vi "SHIFT REGISTER.vi"() -> ()   [LabVIEW 2017]
panel:
  out "X(i-3)":dbl
  out "X(i-2)":dbl
  out "X(i-1)":dbl
  out "X(i)":dbl
  in  "?":bool
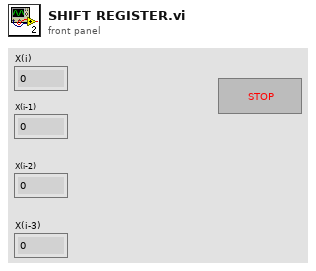
[diagram p1: front panel]
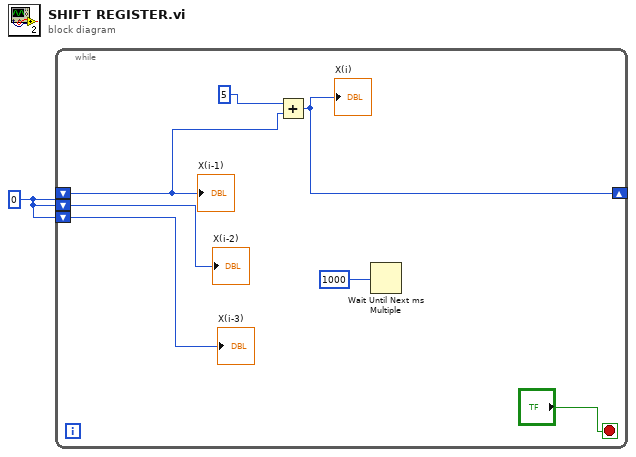
[diagram p0: block diagram]
diagram:
  w1 = 0
  n1 = while {
    shift-right: [w3] -> _
    shift-left: w1 -> [w2]
    shift-left: w1 -> [w6]
    shift-left: w1 -> [w5]
    stop <- "?" stop-if-true
    n2 = Add(x=5, y=w2) -> (x+y=w3:i32)
    "X(i)" <- w3
    n3 = Wait Until Next ms Multiple(millisecond multiple=1000) -> ()  [unwired: 1 out]
    "X(i-3)" <- w5
    "X(i-2)" <- w6
    "X(i-1)" <- w2
  }
